vi "Get ClassType.vi"(8 "error in (no error)":errorcluster, 11 "Message in":refnum<class "Message.lvclass">) -> (0 "error out":errorcluster, 2 "Class Type":string, 3 "Message out":refnum<class "Message.lvclass">)   [LabVIEW 2018, in "LapDog.Messaging.v3.lvlib" / "Message.lvclass"]
doc: "Returns the semantically meaningful [b]namespace[/b] of the message object. This is the fully qualified namespace with the library file extensions (.lvlib, .lvclass) removed.\n\nThis method executes regardless of the error in state."
uses:
  Message.lvclass
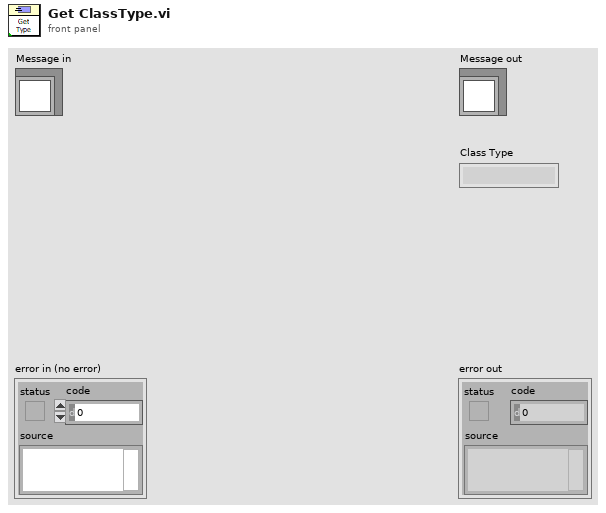
[diagram p1: front panel]
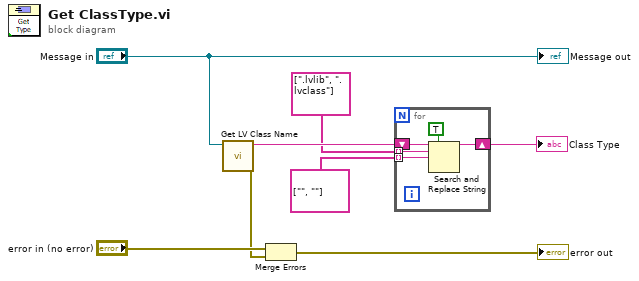
[diagram p0: block diagram]
diagram:
  n1 = call <vilib>:"Get LV Class Name.vi"("object"="Message in") -> ("error out"=w2:errorcluster, "class name"=w8:string)  [unwired: 9 in]
  n2 = Merge Errors("error in (no error)", w2) -> (→"error out":errorcluster)
  n3 = for {
    shift-right: [w11] -> w4
    shift-left: w8 -> [w13]
    tunnel: string[] [".lvlib", ".lvclass"] -> [w10] mode=indexing
    tunnel: string[] ["", ""] -> [w9] mode=indexing
    n4 = Search and Replace String(replace all?=TRUE ("replace all? (F)"), input string=w13, search string=w10, replace string=w9) -> (result string=w11:string)  [unwired: 4 in, 3 out]
  }
  "Class Type" <- w4
  "Message out" <- "Message in"
